vi "Configure Jitter Spectrum.vi"(0 "VISA resource name":refnum<visa-resource-name>, 1 "Enable Jitter Spectrum (T: Enable)":bool=TRUE, 2 "Auto Vertical Mode  (T: Enable)":bool=TRUE, 3 "Jiter Spectrum Vertical Offset (0 s)":dbl, 5 "Window Mode (0: Hanning)":i32(ring) items=["Hanning", "Flat Top", "Rectangular", "Black-Harris", "Hamming"], 7 "Jitter Spectrum Center Frequency (0 Hz)":dbl, 9 "Jitter Spectrum Horizontal Range (10E9 Hz)":dbl=10000000000.0, 11 "error in (no error)":errorcluster, 12 "Auto Horizontal Mode (T: Enable)":bool=TRUE, 13 "Jitter Spectrum Vertical Range (0.01 s)":dbl=0.01) -> (4 "VISA resource name out":refnum<visa-resource-name>, 15 "error out":errorcluster)   [LabVIEW 2020, in "Agilent 90000 Series.lvlib"]
doc: "Configures the jitter spectrum analysis and its parameters."
uses:
  Agilent 90000 Series.lvlib
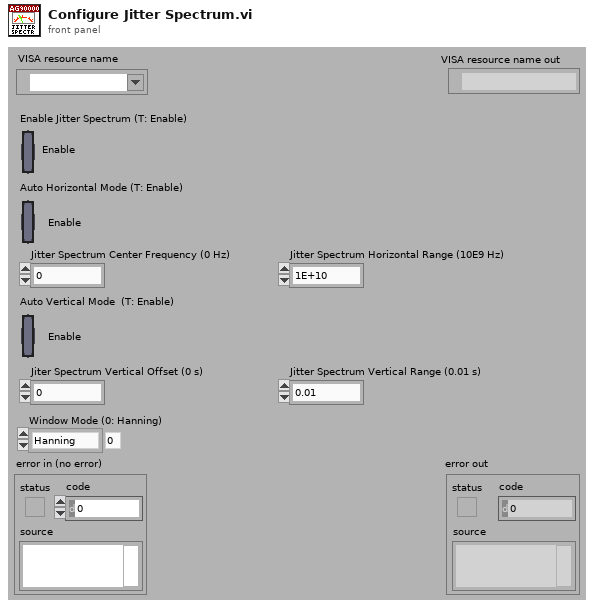
[diagram p1: front panel]
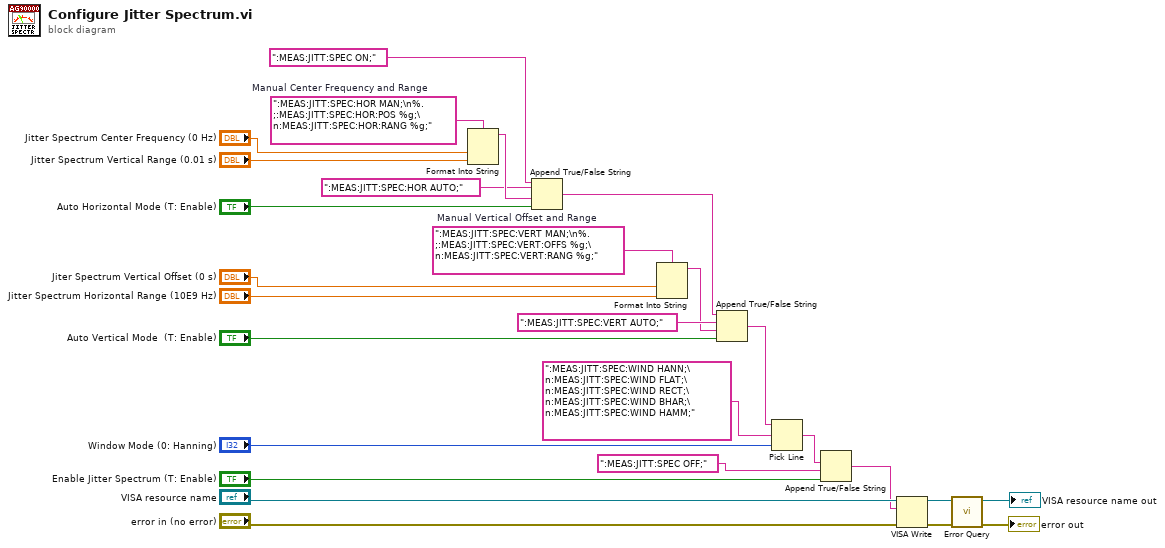
[diagram p0: block diagram]
diagram:
  w17 = ":MEAS:JITT:SPEC:VERT MAN;\n%.;:MEAS:JITT:SPEC:VERT:OFFS %g;\n:MEAS:JITT:SPEC:VERT:RANG %g;"  # Manual Vertical Offset and Range
  w21 = ":MEAS:JITT:SPEC:HOR MAN;\n%.;:MEAS:JITT:SPEC:HOR:POS %g;\n:MEAS:JITT:SPEC:HOR:RANG %g;"  # Manual Center Frequency and Range
  n1 = Format Into String(format string=w21, "Jitter Spectrum Center Frequency (0 Hz)", "Jitter Spectrum Vertical Range (0.01 s)") -> (resulting string=w7:string)  [unwired: 2 in, 1 out]
  n2 = Append True/False String(1:"Auto Horizontal Mode (T: Enable)", 2:w7, 3:":MEAS:JITT:SPEC:HOR AUTO;" ("false string"), 4:":MEAS:JITT:SPEC ON;" ("false string")) -> (0:w5:string)
  n3 = Format Into String(format string=w17, "Jiter Spectrum Vertical Offset (0 s)", "Jitter Spectrum Horizontal Range (10E9 Hz)") -> (resulting string=w6:string)  [unwired: 2 in, 1 out]
  n4 = Append True/False String(1:"Auto Vertical Mode  (T: Enable)", 2:w6, 3:":MEAS:JITT:SPEC:VERT AUTO;" ("true string"), 4:w5) -> (0:w3:string)
  n5 = Pick Line(string ("")=w3, multi-line string=":MEAS:JITT:SPEC:WIND HANN;\n:MEAS:JITT:SPEC:WIND FLAT;\n:MEAS:JITT:SPEC:WIND RECT;\n:MEAS:JITT:SPEC:WIND BHAR;\n:MEAS:JITT:SPEC:WIND HAMM;", line index="Window Mode (0: Hanning)") -> (output string=w2:string)
  n6 = Append True/False String(1:"Enable Jitter Spectrum (T: Enable)", 2:":MEAS:JITT:SPEC OFF;" ("false string"), 3:w2) -> (0:w9:string)  [unwired: 1 out]
  n7 = VISA Write(VISA resource name="VISA resource name", write buffer=w9, error in (no error)="error in (no error)") -> (VISA resource name out=w25:refnum<visa-resource-name>, error out=w24:errorcluster)  [unwired: 1 out]
  n8 = call "Error Query.vi"("error in (no error)"=w24, "VISA resource name"=w25) -> ("error out"=→"error out":errorcluster, "VISA resource name out"=→"VISA resource name out":refnum<visa-resource-name>)  [unwired: 8 out]
